vi "as2_startLogFile.vi"(4 "error in (no error)":errorcluster, 6 "Path In":path) -> (0 "error out":errorcluster, 2 "Path":path)   [LabVIEW 2009]
uses:
  <vilib>/Utility/file.llb/Write To Spreadsheet File (string).vi
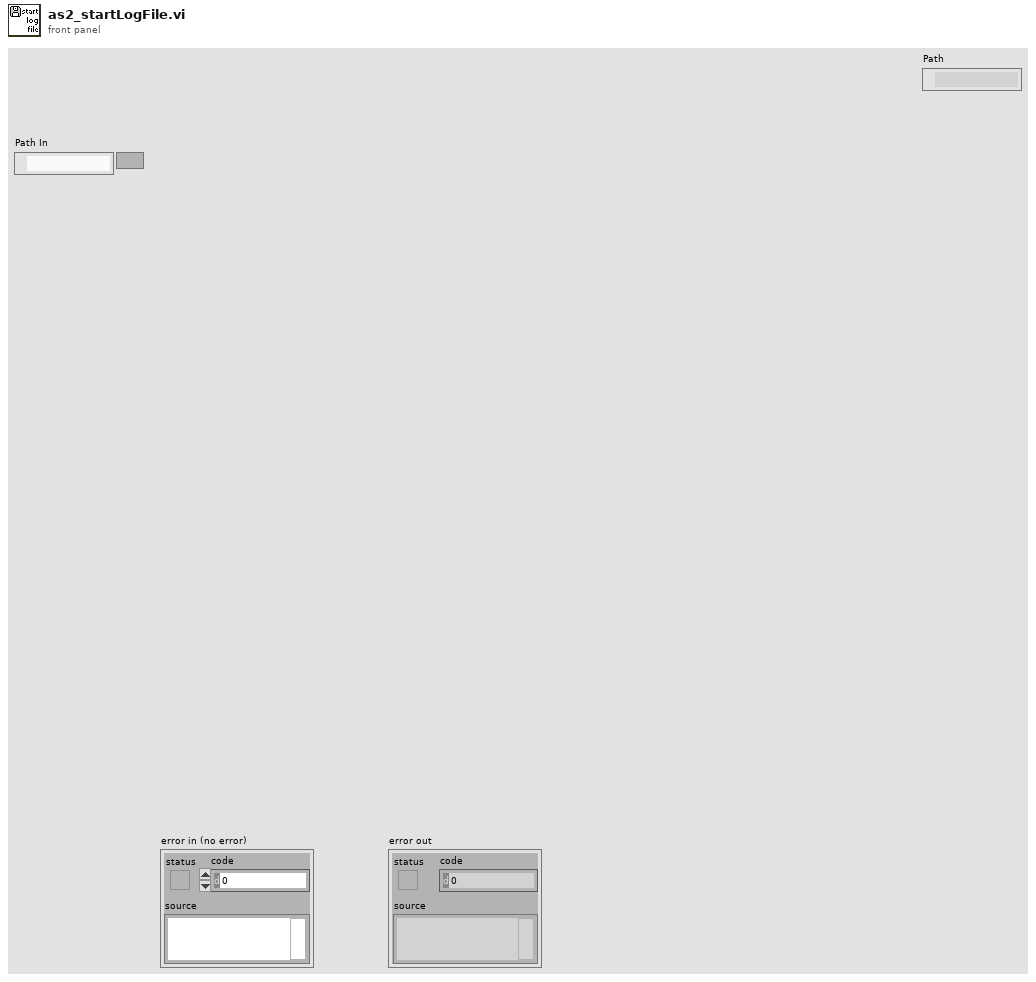
[diagram p1: front panel]
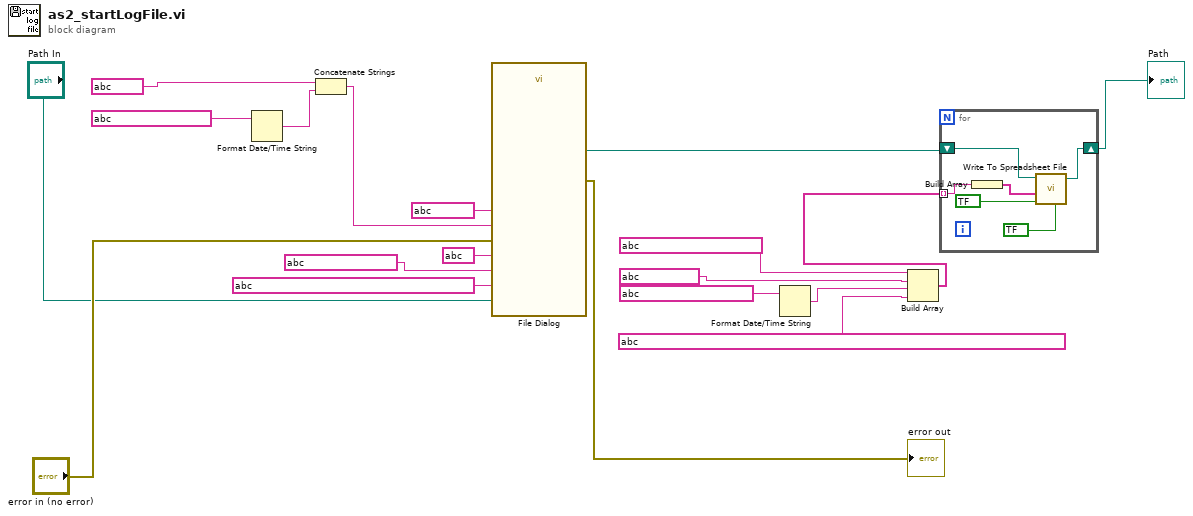
[diagram p0: block diagram]
diagram:
  n1 = Format Date/Time String(time format string (%c)=string ?) -> (date/time string=w14:string)  [unwired: 2 in]
  n2 = Concatenate Strings(string ?, w14) -> (w13:string)
  n3 = call "File Dialog"("start path"="Path In", "prompt"=string ?, "button label"=string ?, "default name"=w13, "error in"="error in (no error)", "pattern (all files)"=string ?, "pattern label"=string ?) -> ("selected path"=w2:path, "error out"=→"error out":errorcluster)  [unwired: 5 in, 2 out]
  n4 = Format Date/Time String(time format string (%c)=string ?) -> (date/time string=w4:string)  [unwired: 2 in]
  n5 = Build Array(string ?, string ?, w4, string ?) -> (w5:string[])
  n6 = for {
    tunnel: w5 -> [w22] mode=indexing
    shift-right: [w24] -> w1
    shift-left: w2 -> [w23]
    n7 = Build Array(w22) -> (w21:string[])
    n8 = call-poly <vilib>:"Write To Spreadsheet File.vi"("transpose? (no:F)"=bool ?, "append to file? (new file:F)"=bool ?, "1D data"=w21, "file path (dialog if empty)"=w23) -> ("new file path (Not A Path if cancelled)"=w24:path)  [unwired: 4 in]
  }
  "Path" <- w1
